vi "Get data time.vi"(1 "sampling info":cluster{"Fs":dbl, "#s":dbl}) -> (0 "Array":dbl[](array[numeric]) format="%#_6f")   [LabVIEW 2013]
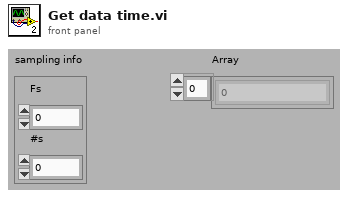
[diagram p1: front panel]
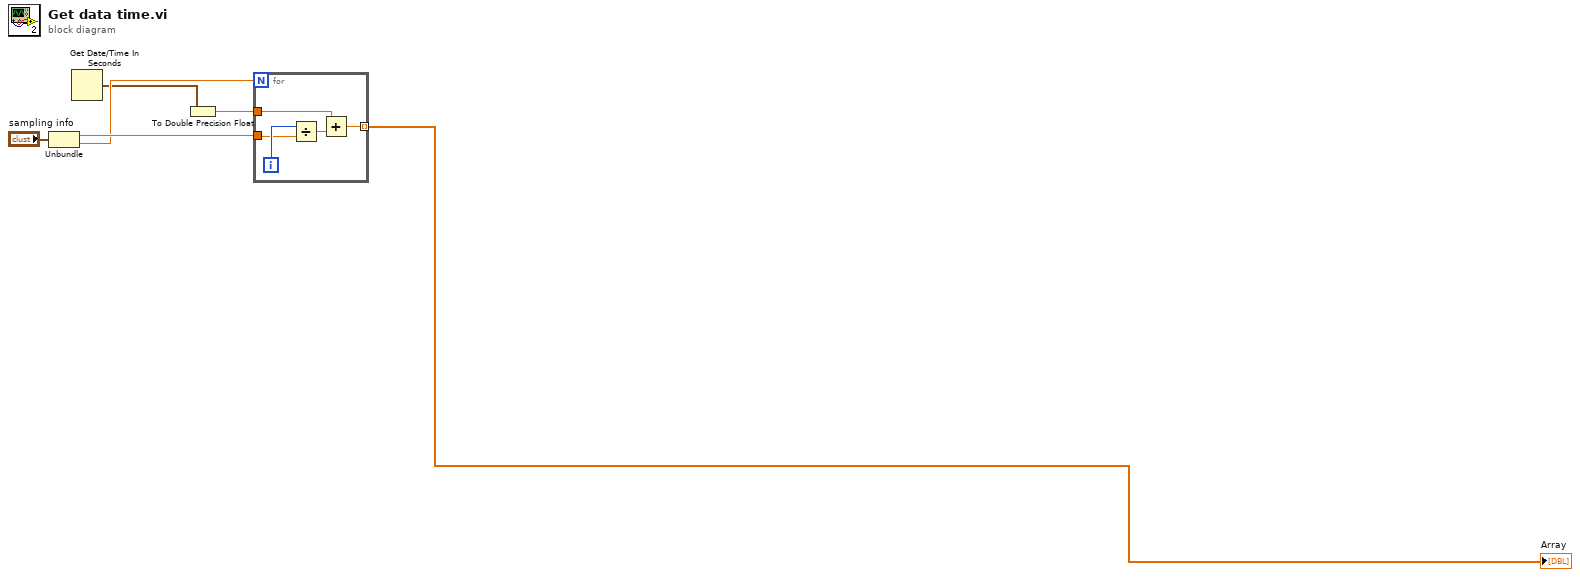
[diagram p0: block diagram]
diagram:
  n1 = Unbundle("sampling info") -> ("Fs"=w4:dbl, "#s"=w3:dbl)
  n2 = Get Date/Time In Seconds() -> (seconds since 1Jan1904=w1:timestamp)
  n3 = To Double Precision Float(number=w1) -> (double precision float=w5:dbl)
  n4 = for {
    N: w3 -> [_]
    tunnel: w4 -> [w10]
    tunnel: w5 -> [w8]
    tunnel: [w7] -> w6 mode=indexing
    i -> [w11]
    n5 = Divide(x=w11, y=w10) -> (x/y=w9:dbl)
    n6 = Add(x=w8, y=w9) -> (x+y=w7:dbl)
  }
  "Array" <- w6
